vi "Archive Files.vi"(8 "error in (no error)":errorcluster, 10 "pattern":string="*.xml", 11 "Folder Path":path) -> (0 "error out":errorcluster)   [LabVIEW 2013, in "Utilities 1.lvlib"]
uses:
  Utilities 1.lvlib
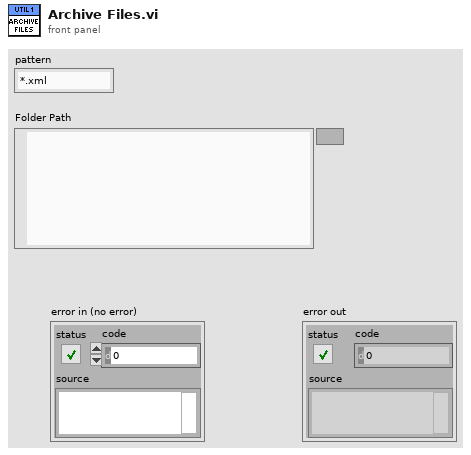
[diagram p1: front panel]
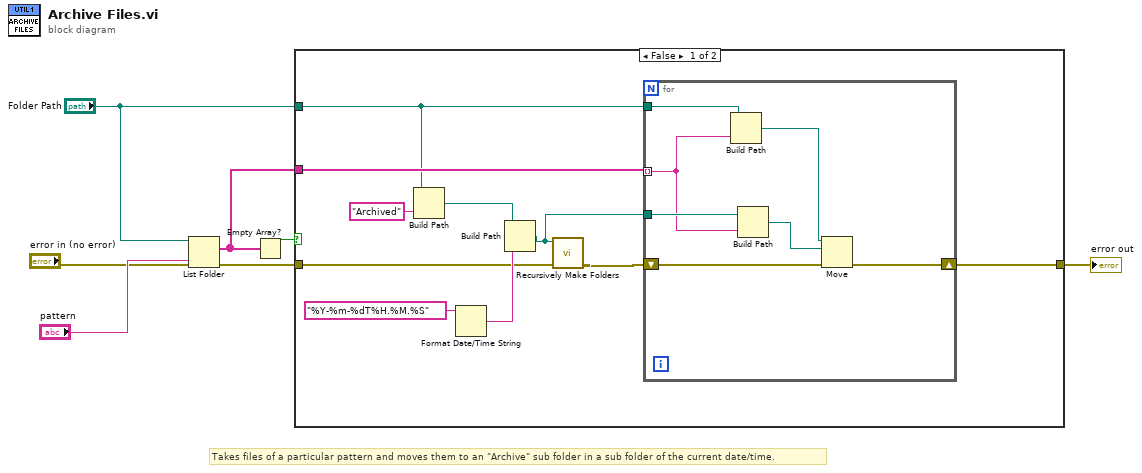
[diagram p0: block diagram]
diagram:
  # "Takes files of a particular pattern and moves them to an \"Archive\" sub folder in a sub folder of the current date/time."
  n1 = List Folder(path="Folder Path", pattern="pattern", error in="error in (no error)") -> (filenames=w4:string[], error out=w6:errorcluster)  [unwired: 1 in, 2 out]
  n2 = Empty Array?(array=w4) -> (empty?=w5:bool)
  n3 = case shown="False" w5 {
    tunnel: w6 -> [w12 w25]
    tunnel: w4 -> [w17 _]
    tunnel: "Folder Path" -> [w10 _]
    tunnel: [w8 w25] -> w1
    frame False {
      n4 = Build Path(base path=w10, name or relative path="Archived") -> (appended path=w15:path)
      n5 = Format Date/Time String(time format string (%c)="%Y-%m-%dT%H.%M.%S") -> (date/time string=w13:string)  [unwired: 2 in]
      n6 = Build Path(base path=w15, name or relative path=w13) -> (appended path=w9:path)
      n7 = call "Recursively Make Folders.vi"("error in (no error)"=w12, "directory path"=w9) -> ("error out"=w11:errorcluster)  [unwired: 4 in, 1 out]
      n8 = for {
        tunnel: w17 -> [w21] mode=indexing
        tunnel: w10 -> [w24]
        tunnel: w9 -> [w22]
        shift-right: [w18] -> w8
        shift-left: w11 -> [w19]
        n9 = Build Path(base path=w24, name or relative path=w21) -> (appended path=w23:path)
        n10 = Build Path(base path=w22, name or relative path=w21) -> (appended path=w20:path)
        n11 = Move(source path=w23, error in=w19, 10:w20) -> (error out=w18:errorcluster)  [unwired: 2 in, 2 out]
      }
    }
    frame True {
    }
  }
  "error out" <- w1
